vi "Read CAN Settings from DB.vi"(8 "error in":errorcluster, 10 "ECU CAN Port":string, 11 "Socket No":u16) -> (0 "error out":errorcluster, 3 "Read CAN Setting":T3 {"CAN Init Data"."scope (normal)" items=["Normal", "Session Only", "Interface Only", "Session Only Blocking"]; "CAN Init Data"."CAN:Termination" items=["Off", "On"]; "CAN Init Data"."Baud Rate" format="%.0p"})   [LabVIEW 2023, in "LTT_TeststandSteptypes.lvlib"]
uses:
  LTT_TeststandSteptypes.lvlib
  HardwareAbstractionLayer_LVOOP/CAN/CAN Lib/CAN_class/Ctrls/CAN Init Ctrl.ctl
  <vilib>/xnet/xnet.llb/XNET Control Scope.ctl
  HardwareAbstractionLayer_LVOOP/CAN/CAN Lib/CAN_class/CAN.lvclass
  HardwareAbstractionLayer_LVOOP/Database/Database.lvclass
  HardwareAbstractionLayer_LVOOP/Database/SQL Public VI/Control/DB Options.ctl
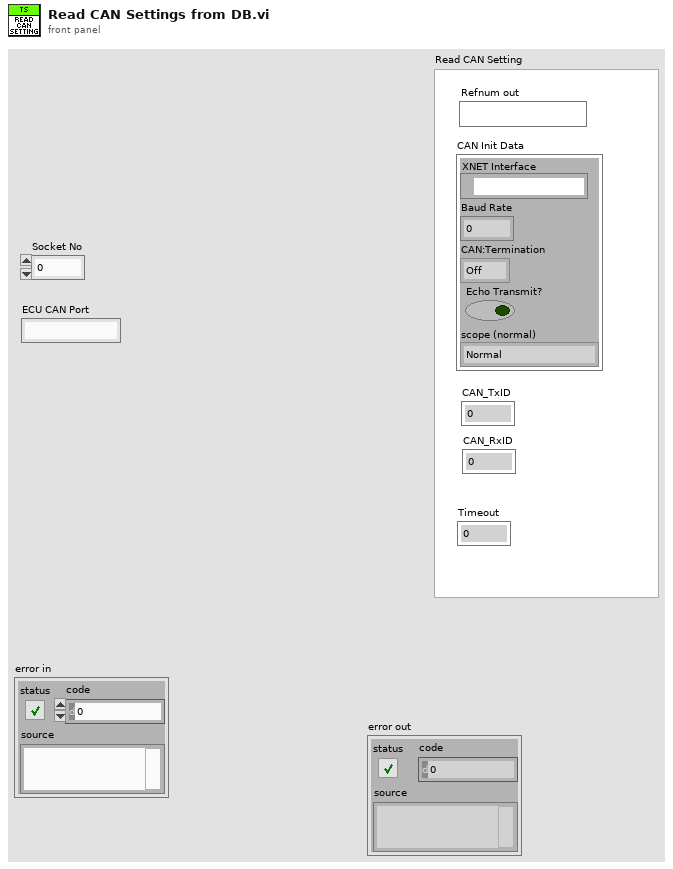
[diagram p1: front panel]
types:
  T1 = typedef "HardwareAbstractionLayer_LVOOP.lvlib/CAN HAL Lib.lvlib/CAN.lvclass/CAN Init Ctrl.ctl" = cluster{"XNET Interface":refnum<k21>, "Baud Rate":u64, "CAN:Termination":u32, "Echo Transmit?":bool, "scope (normal)":T2}
  T2 = typedef "XNET Control Scope.ctl" = u32
  T3 = cluster{"Refnum out":refnum<k21>, "CAN Init Data":T1, "CAN_RxID":u32, "CAN_TxID":u32, "Timeout":dbl}
  T4 = typedef "HardwareAbstractionLayer_LVOOP.lvlib/Database.lvclass/DB Options.ctl" = enum16{"Init", "Select Data", "Insert Data", "Update Data", "Delete Data", "Execute Query", "Create Schema", "Create Table", "List Tables", "List Columns", "Close"}
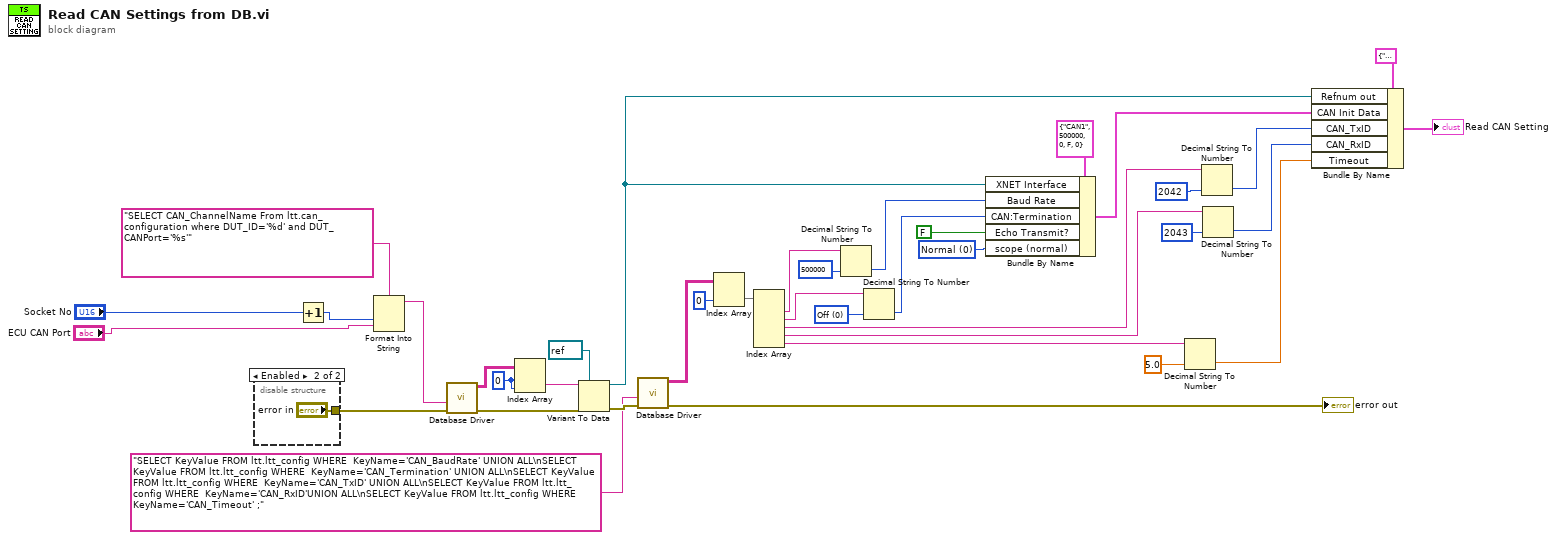
[diagram p0: block diagram]
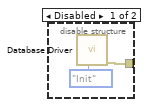
[diagram p2: hidden frame]
diagram:
  w1 = T2 0 items=["Normal", "Session Only", "Interface Only", "Session Only Blocking"] ("scope (normal)")
  w33 = u32 0 items=["Off", "On"] ("CAN:Termination")
  w19 = 0 ("index (row)")
  n1 = disable-structure shown="Enabled" {
    disable-tunnel: [w41 "error in"] -> w13
    frame Disabled {
      n2 = call "Database Driver.vi"("Options"=DB_Options."Init") -> ("error out"=w41:errorcluster)  [unwired: 7 in, 3 out]
    }
    frame Enabled {
    }
  }
  n3 = Increment(x="Socket No") -> (x+1=w16:u16)
  n4 = Format Into String(format string="SELECT CAN_ChannelName From ltt.can_configuration where DUT_ID='%d' and DUT_CANPort='%s'" ("SQL query"), w16, "ECU CAN Port") -> (resulting string=w14:string)  [unwired: 2 in, 1 out]
  n5 = call "Database Driver.vi"("error in"=w13, "SQL query"=w14) -> ("error out"=w22:errorcluster, "data"=w18:string[][])  [unwired: 6 in, 2 out]
  n6 = Index Array(array=w18, index (row)=w19, index (col)=w19) -> (element=w21:string)
  n7 = Variant To Data(error in=w22, type=refnum<k21> refnum ("XNET Interface"), Variant=w21) -> (data=w7:refnum<k21>, error out=w24:errorcluster)
  n8 = call "Database Driver.vi"("error in"=w24, "SQL query"="SELECT KeyValue FROM ltt.ltt_config WHERE  KeyName='CAN_BaudRate' UNION ALL\nSELECT KeyValue FROM ltt.ltt_config WHERE  KeyName='CAN_Termination' UNION ALL\nSELECT KeyValue FROM ltt.ltt_config WHERE  KeyName='CAN_TxID' UNION ALL\nSELECT KeyValue FROM ltt.ltt_config WHERE  KeyName='CAN_RxID'UNION ALL\nSELECT KeyValue FROM ltt.ltt_config WHERE  KeyName='CAN_Timeout' ;") -> ("error out"=→"error out":errorcluster, "data"=w26:string[][])  [unwired: 6 in, 2 out]
  n9 = Index Array(array=w26, index (col)=0 ("disabled index (col)")) -> (element=w28:string[])  [unwired: 1 in]
  n10 = Index Array(array=w28) -> (element #1=w29:string, element #2=w32:string, element #3=w35:string, element #4=w36:string, element #5=w10:string)  [unwired: 5 in]
  n11 = Decimal String To Number(string=w29, default (0L)=u64 500000 ("Baud Rate")) -> (number=w31:u64)  [unwired: 1 in, 1 out]
  n12 = Decimal String To Number(string=w32, default (0L)=w33) -> (number=w34:u32)  [unwired: 1 in, 1 out]
  n13 = Bundle By Name(cluster=T1 {"XNET Interface"="CAN1", "Baud Rate"=500000, "CAN:Termination"=0, "Echo Transmit?"=FALSE, "scope (normal)"=0} ("CAN Init Data"), "XNET Interface"=w7, "Baud Rate"=w31, "CAN:Termination"=w34, "Echo Transmit?"=FALSE, "scope (normal)"=w1) -> (w8:T1)
  n14 = Decimal String To Number(string=w10, default (0L)=5.0 ("ResponseTimeout (S)")) -> (number=w4:dbl)  [unwired: 1 in, 1 out]
  n15 = Decimal String To Number(string=w35, default (0L)=u32 2042 ("TxID")) -> (number=w6:u32)  [unwired: 1 in, 1 out]
  n16 = Decimal String To Number(string=w36, default (0L)=u32 2043 ("TxID")) -> (number=w5:u32)  [unwired: 1 in, 1 out]
  n17 = Bundle By Name(cluster=T3 {"Refnum out"="", "CAN Init Data"={"XNET Interface"="", "Baud Rate"=0, "CAN:Termination"=0, "Echo Transmit?"=FALSE, "scope (normal)"=0}, "CAN_RxID"=0, "CAN_TxID"=0, "Timeout"=0.0} ("Read CAN Setting"), "Refnum out"=w7, "CAN Init Data"=w8, "CAN_TxID"=w6, "CAN_RxID"=w5, "Timeout"=w4) -> (→"Read CAN Setting":T3)
